vi "Config - RVHR reporting settings.vi"(5 ".ini Controller":enum16{"Read", "Write"}(ring), 7 ".ini filename":string="supervisoryconfig.ini", 8 "error in (no error)":errorcluster, 10 "RVHR Config Cluster In":T1, 11 "Directory Path":path) -> (0 "error out":errorcluster, 1 "appended path":path, 2 "RVHR Config Cluster Out":T1)   [LabVIEW 2023]
doc: "Obtains default hlc configuration information from an .ini file"
uses:
  <vilib>/Utility/config.llb/NI_LVConfig.lvlib
  Controls/RVHR - Reporting Settings.ctl
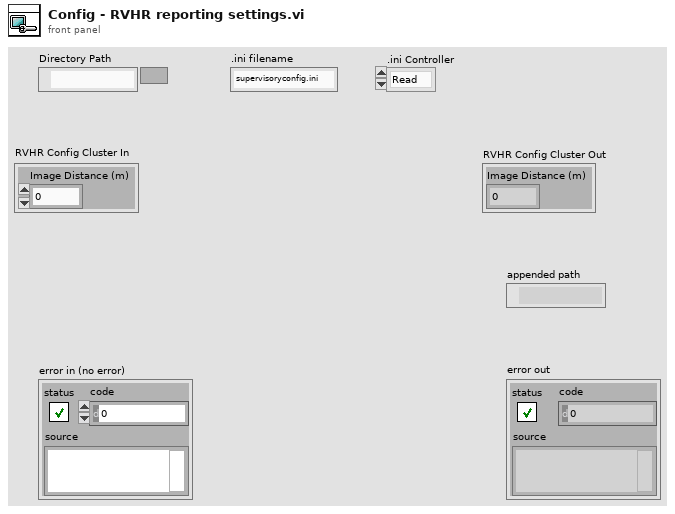
[diagram p1: front panel]
types:
  T1 = typedef "RVHR - Reporting Settings.ctl" = cluster{"Image Distance (m)":dbl}
  T2 = typedef "NI_LVConfig.lvlib/Config Data RefNum.ctl" = refnum<k1>
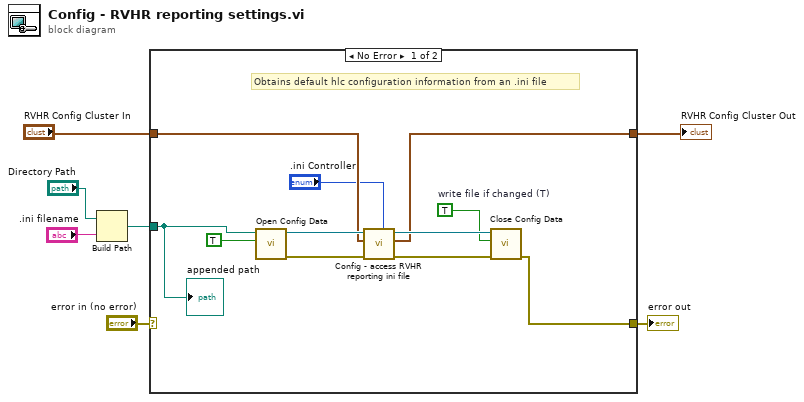
[diagram p0: block diagram]
diagram:
  n1 = Build Path(base path="Directory Path", name or relative path=".ini filename") -> (appended path=w5:path)
  n2 = case shown="No Error" "error in (no error)" {
    selector: "error in (no error)" -> [_ w19]
    tunnel: [w12 _] -> w1
    tunnel: [w11 w19] -> w6
    tunnel: w5 -> [w10 _]
    tunnel: "RVHR Config Cluster In" -> [w9 _]
    frame No Error {
      w14 = TRUE  # write file if changed (T)
      # "Obtains default hlc configuration information from an .ini file"
      n3 = call <vilib>:"Open Config Data.vi"("create file if necessary (T)"=TRUE, "configuration file path"=w10) -> ("error out"=w17:errorcluster, "refnum"=w15:T2)  [unwired: 7 in, 1 out]
      n4 = call "Config - access RVHR reporting ini file.vi"(".ini Controller"=".ini Controller", "error in"=w17, "RVHR Settings"=w9, "Config File Ref"=w15) -> ("error out"=w18:errorcluster, "HLC Controls Out"=w12:T1, "refnum out"=w16:T2)  [unwired: 5 in]
      n5 = call <vilib>:"Close Config Data.vi"("error in (no error)"=w18, "write file if changed (T)"=w14, "refnum"=w16) -> ("error out"=w11:errorcluster)  [unwired: 7 in, 1 out]
      "appended path" <- w10
    }
    frame Error {
    }
  }
  "error out" <- w6
  "RVHR Config Cluster Out" <- w1
